vi "nanocal-frontend-18.vi"() -> ()   [LabVIEW 2018]
uses:
  nanocal - config.ctl
  resistoricicle.ctl
  channelicicle.ctl
  nanocal/Nanocalorimetry/data/MCL.lvlibp/SynkTek FPGA/FPGA_SharedResources/FPGASharedResources_Readings_ReadingChannelTypedef.ctl
  nanocal/Nanocalorimetry/data/MCL.lvlibp/SynkTek FPGA/FPGA_SharedResources/FPGASharedResources_Lockin_Typedef.ctl
  agregator -- action.ctl
  publisher action.ctl
  nanocal calc command.ctl
  copy of gyro pll V3 for LV18/cursor action.ctl
  linear interpolation iiii- complex.vi
  nanocal/Nanocalorimetry/data/NanoCalLib.lvlibp
  nanocal/Nanocalorimetry/data/MCL.lvlibp/SynkTek FPGA/FPGA_SharedResources/FPGA_SharedResources.lvlib
panel:
  in  "wait (ms)":u32=30
  in  "Stop":bool
  in  "Tab Control 2":enum32{"config", "read", "plots"}(tab)
  in  "nanocal config":T1={"Hs"={"out"=enum."D", "shunt R (Ohm)"=100000.0, "V"={"c"=enum."A V1", "l"=enum."Lock-in set L1"}, "\"I\""={"c"=enum."A V2", "l"=enum."Lock-in set L1"}}, "ofset heater"={"out"=enum."C", "\"I\""=enum."C V2", "shunt R (Ohm)"=10000.0}, "Ts"={"out"=enum."D", "shunt R (Ohm)"=100000.0, "V"={"c"=enum."D V1", "l"=enum."Lock-in set L1"}, "\"I\""={"c"=enum."D V2", "l"=enum."Lock-in set L1"}}, "Tr"={"out"=enum."B", "shunt R (Ohm)"=100000.0, "V"={"c"=enum."E V1", "l"=enum."Lock-in set L1"}, "\"I\""={"c"=enum."E V2", "l"=enum."Lock-in set L1"}}, "Hr"={"out"=enum."E", "shunt R (Ohm)"=100000.0, "V"={"c"=enum."B V1", "l"=enum."Lock-in set L1"}, "\"I\""={"c"=enum."B V2", "l"=enum."Lock-in set L1"}}, "differential"={"c"=enum."C V1", "l"=enum."Lock-in set L2"}} {"Hr"."shunt R (Ohm)" format="%#_6p"; "Tr"."shunt R (Ohm)" format="%#_6p"; "Ts"."shunt R (Ohm)" format="%#_6p"; "ofset heater"."shunt R (Ohm)" format="%#_6p"; "Hs"."shunt R (Ohm)" format="%#_6p"}
  out "diff":cluster{dbl[], dbl[]}[](graph)
  in  "history size":i32=10000
  out "C (J/K)":cluster{dbl[], dbl[]}[](graph)
  out "Ts":cluster{dbl[], dbl[]}[](graph)
  out "R(omega)":cluster{dbl[], dbl[]}[](graph)
  out "1/R(omega)":cluster{dbl[], dbl[]}[](graph)
  out "frequency (Hz)":dbl format="%#_3p"
  out "Cs (J/K)":dbl format="%#_3p"
  out "Ks (W/K)":dbl format="%#_3p"
  out "Hs -- \"I\" (V)":cdb format="%#_3p"
  out "Ts -- \"I\" (V)":cdb format="%#_3p"
  out "Ts":dbl format="%#_3p"
  # "Ts"
  # "Tr"
  # "Hs"
  # "Hr"
  # "offset heater"
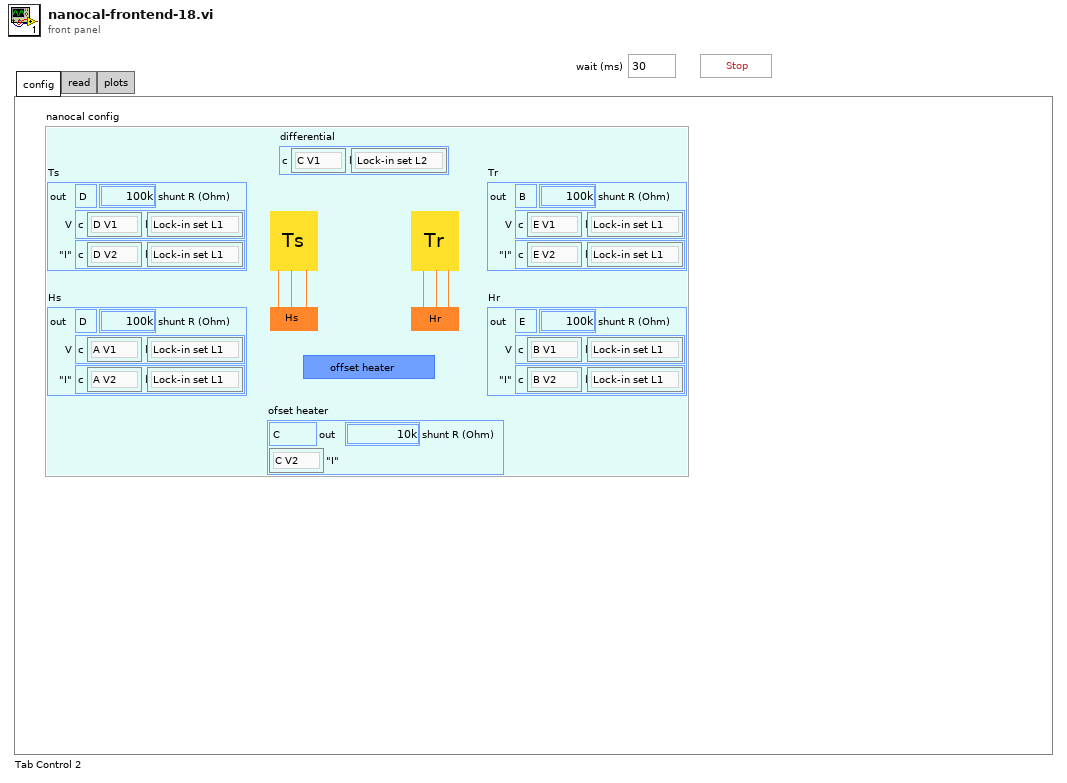
[diagram p1: front panel]
types:
  T1 = typedef "nanocal - config.ctl" = cluster{"Hs":T2, "ofset heater":cluster{"out":enum16{"A", "B", "C", "D", "E"}, "\"I\"":T4, "shunt R (Ohm)":dbl}, "Ts":T2, "Tr":T2, "Hr":T2, "differential":T3}
  T2 = typedef "resistoricicle.ctl" = cluster{"out":enum16{"A", "B", "C", "D", "E"}, "shunt R (Ohm)":dbl, "V":T3, "\"I\"":T3}
  T3 = typedef "channelicicle.ctl" = cluster{"c":T4, "l":T5}
  T4 = typedef "MCL.lvlibp/FPGA_SharedResources.lvlib/FPGASharedResources_Readings_ReadingChannelTypedef.ctl" = enum8{"A V1", "A V2", "B V1", "B V2", "C V1", "C V2", "D V1", "D V2", "E V1", "E V2", "A I", "B I", "C I", "D I", "E I", "Int."}
  T5 = typedef "MCL.lvlibp/FPGA_SharedResources.lvlib/FPGASharedResources_Lockin_Typedef.ctl" = enum8{"Lock-in set L1", "Lock-in set L2"}
  T6 = typedef "agregator -- action.ctl" = enum16{"append", "interpolate", "empty!", "force", "init", "scale", "read last"}
  T7 = typedef "MCL.lvlibp/MCL_DataRef.ctl" = refnum<vi>
  T8 = typedef "cursor action.ctl" = enum16{"range", "read", "write", "check", "zoom out", "smart zoom out", "zoom to aspect ratio 1", "zoom to win", "zoom out 20%", "zoom in 20%", "-empty", "smart zoom out&aspect", "move range left 20%", "move range right 20%", "move range up 20%", "move range down 20%", "zoom to X win", "zoom to Y win", "zoom out X", "zoom out Y", "zoom in X", "zoom in Y", "check plot scale"}
  T9 = typedef "nanocal calc command.ctl" = enum16{"void", "R(omega)", "C/T (J/K^2)"}
  T10 = typedef "publisher action.ctl" = enum16{"set", "get", "init", "check"}
  T11 = typedef "engine reading icicle.ctl" = cluster{"Ts -- V (V)":cdb, "Hr -- V (V)":cdb, "Hs -- V (V)":cdb, "Tr -- V (V)":cdb, "Diff -- V (V)":cdb, "offset (V)":cdb, "Ts -- \"I\" (V)":cdb, "Hs -- \"I\" (V)":cdb, "Tr -- \"I\" (V)":cdb, "Hr -- \"I\" (V)":cdb, "freq (Hz)":dbl}
  T12 = typedef "icicle.ctl" = cluster{"name":string, "units":string, "data":dbl}
  T13 = typedef "interpolation state - complex.ctl" = cluster{"requested size":i32, "Array":cdb[], "actual number of elements":i32}
  T14 = typedef "eventvkey.ctl" = enum16{"ASCII", "Enter", "Return", "Shift", "Ctrl", "Alt", "Cmd", "Opt", "Caps", "NumLock", "Clear", "Break", "Up", "Down", "Left", "Right", "Insert", "Delete", "Home", "End", "PageUp", "PageDown", "Escape", "Help", "Pause", "ScrollLock", "F1", "F2", "F3", "F4", "F5", "F6", "F7", "F8", "F9", "F10", "F11", "F12", "F13", "F14", "F15", "F16", "F17", "F18", "F19", "F20", "F21", "F22", "F23", "F24", "Play", "VolumeUp", "VolumeDown", "Mute", "Two Byte Char"}
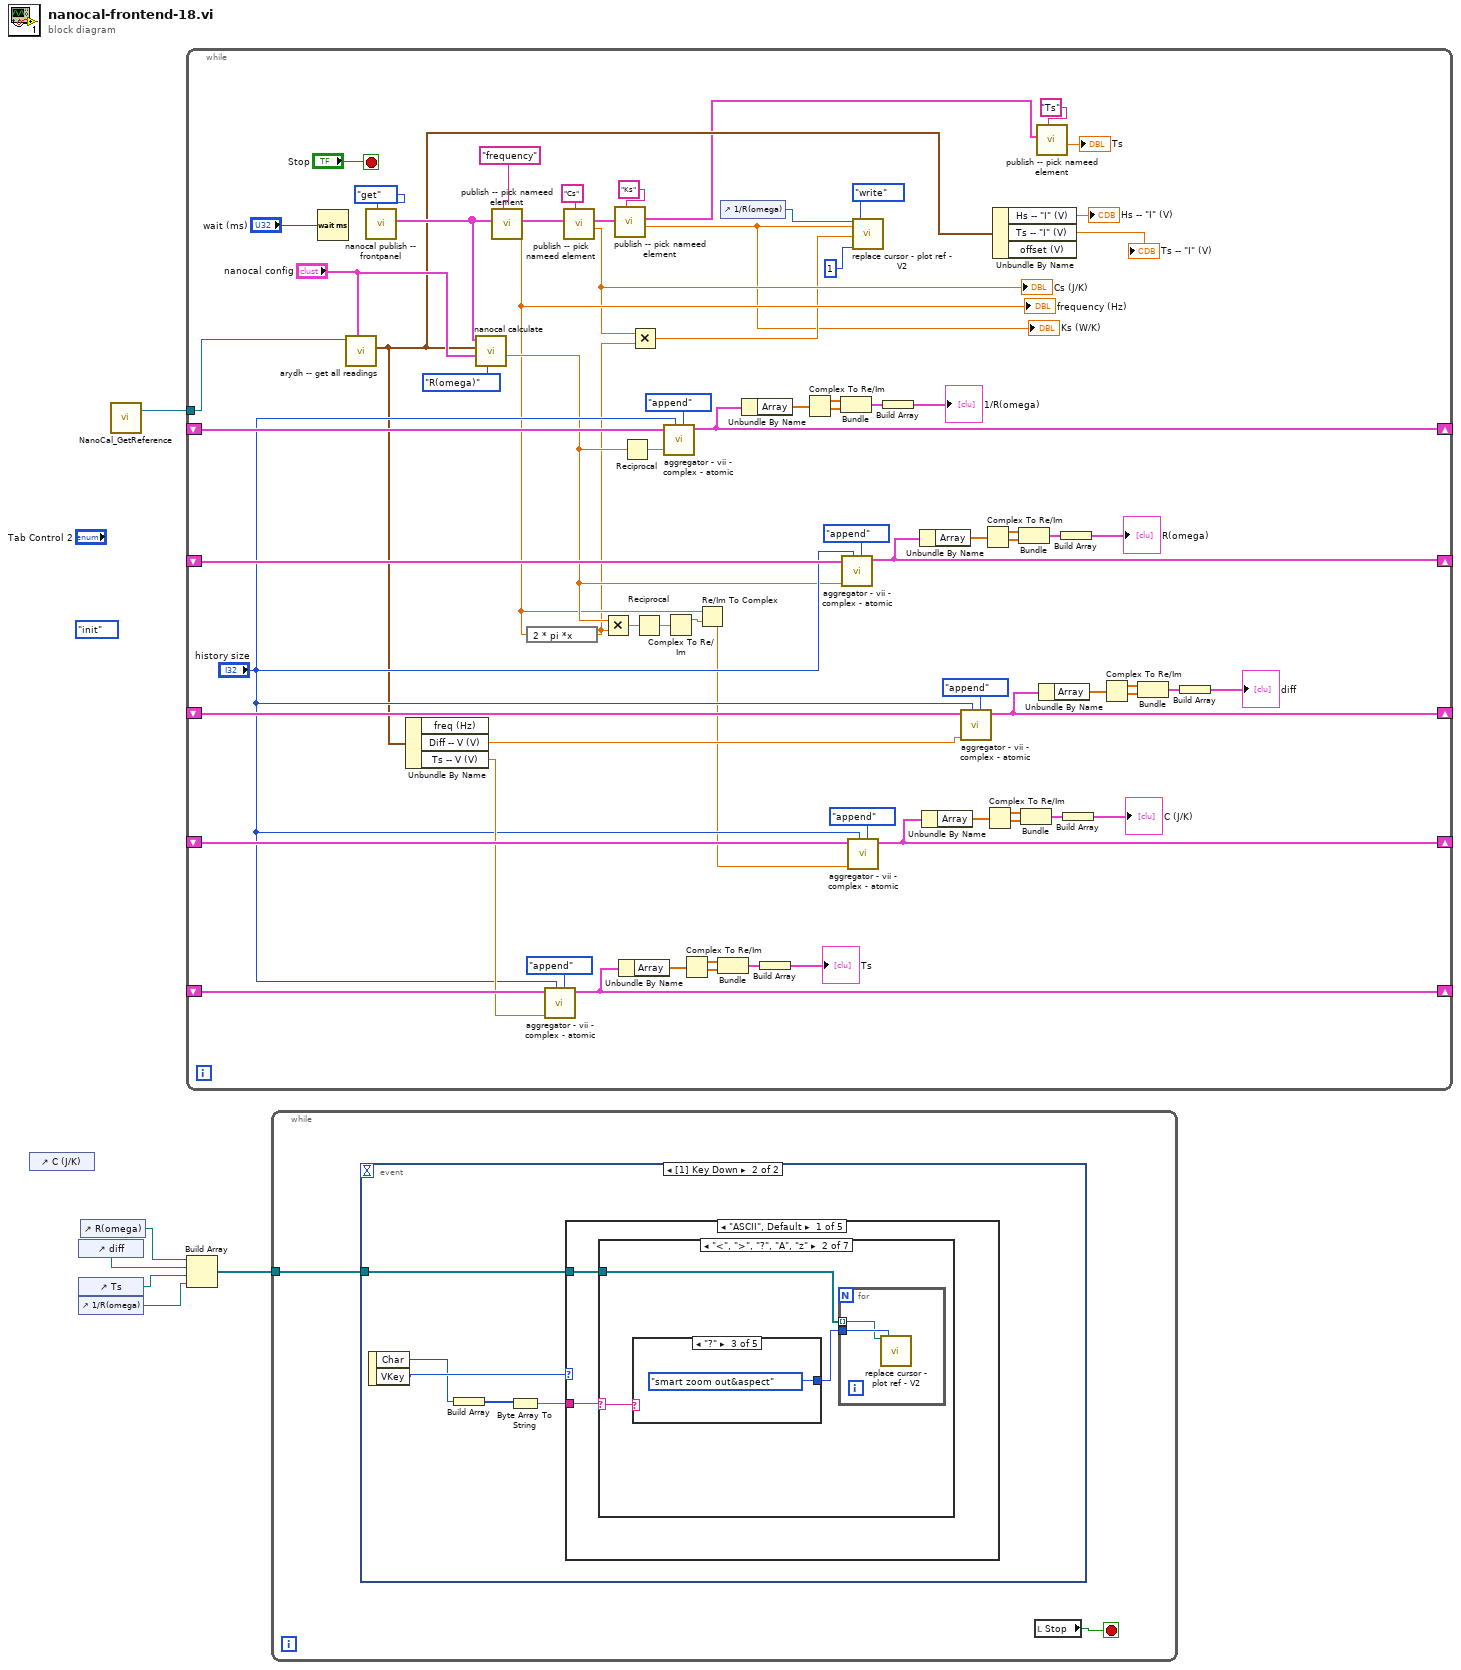
[diagram p0: block diagram]
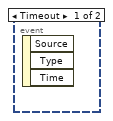
[diagram p2: hidden frame]
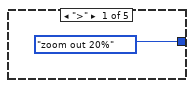
[diagram p4: hidden frame]
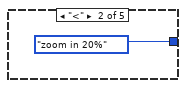
[diagram p5: hidden frame]
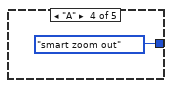
[diagram p6: hidden frame]
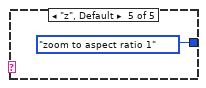
[diagram p7: hidden frame]
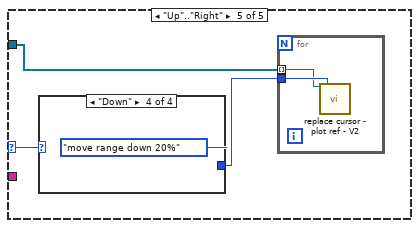
[diagram p16: hidden frame]
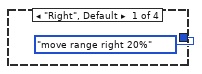
[diagram p17: hidden frame]
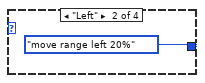
[diagram p18: hidden frame]
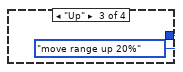
[diagram p19: hidden frame]
diagram:
  (unwired) agregator_--_action."init" ("aggregator action")
  n1 = control-ref of="C (J/K)"() -> ()  [unwired: 1 out]
  n2 = control-ref of="diff"() -> (w3:refnum<vi>)
  n3 = control-ref of="Ts"() -> (w4:refnum<vi>)
  n4 = control-ref of="1/R(omega)"() -> (w5:refnum<vi>)
  n5 = control-ref of="R(omega)"() -> (w1:refnum<vi>)
  n6 = call "NanoCal_GetReference.vi"() -> ("Connected MCL object"=w6:T7)  [unwired: 2 in, 1 out]
  n7 = while {
    tunnel: w6 -> [w47]
    shift-right: [w77] -> _
    shift-left: _ -> [w79]
    shift-right: [w65] -> _
    shift-left: _ -> [w64]
    shift-right: [w57] -> _
    shift-left: _ -> [w56]
    shift-right: [w49] -> _
    shift-left: _ -> [w48]
    shift-right: [w35] -> _
    shift-left: _ -> [w34]
    stop <- "Stop" stop-if-true
    n8 = Wait (ms)(milliseconds to wait="wait (ms)") -> ()  [unwired: 1 out]
    n9 = call "arydh -- get all readings.vi"("nanocal config"="nanocal config", "MCL object"=w47) -> ("engine reading"=w12:T11)  [unwired: 9 in]
    n10 = call "nanocal publish -- frontpanel.vi"("publisher action"=publisher_action."get") -> ("nanocal data array OUT"=w24:T12[])  [unwired: 10 in]
    n11 = Unbundle By Name(w12) -> ("Diff -- V (V)"=w46:cdb, "Ts -- V (V)"=w45:cdb)  [unwired: 1 out]
    n12 = call "nanocal calculate.vi"("nanocal calc command"=nanocal_calc_command."R(omega)", "nanocal config"="nanocal config", "engine reading"=w12, "nanocal data array"=w24) -> ("number"=w31:cdb)  [unwired: 7 in]
    n13 = call "publish -- pick nameed element.vi"("name"="frequency", "nanocal data array"=w24) -> ("element"=w26:dbl, "nanocal data array OUT"=w16:T12[])  [unwired: 8 in]
    "frequency (Hz)" <- w26
    n14 = expression code="2 * pi *x"(w26) -> (w22:dbl)
    n15 = call "aggregator - vii - complex - atomic.vi"("aggregator action"=agregator_--_action."append", "requested size"="history size", "number"=w45, "state IN"=w56) -> ("state OUT"=w57:T13)  [unwired: 4 in, 3 out]
    n16 = call "publish -- pick nameed element.vi"("name"="Cs", "nanocal data array"=w16) -> ("element"=w21:dbl, "nanocal data array OUT"=w23:T12[])  [unwired: 8 in]
    "Cs (J/K)" <- w21
    n17 = Multiply(x=w31, y=w22) -> (x*y=w30:cdb)
    n18 = call "publish -- pick nameed element.vi"("name"="Ks", "nanocal data array"=w23) -> ("element"=w19:dbl, "nanocal data array OUT"=w8:T12[])  [unwired: 8 in]
    "Ks (W/K)" <- w19
    n19 = Unbundle By Name(w57) -> ("Array"=w62:cdb[])
    n20 = Reciprocal(x=w31) -> (1/x=w32:cdb)
    n21 = Multiply(x=w21, y=w22) -> (x*y=w20:dbl)
    n22 = Reciprocal(x=w30) -> (1/x=w29:cdb)
    n23 = call "aggregator - vii - complex - atomic.vi"("aggregator action"=agregator_--_action."append", "requested size"="history size", "number"=w32, "state IN"=w34) -> ("state OUT"=w35:T13)  [unwired: 4 in, 3 out]
    n24 = Complex To Re/Im(x + iy=w29) -> (x=w28:dbl)  [unwired: 1 out]
    n25 = Complex To Re/Im(x + iy=w62) -> (x=w61:dbl[], y=w60:dbl[])
    n26 = Re/Im To Complex(1:w28, 2:w26) -> (0:w27:cdb)
    n27 = Bundle(w61, w60) -> (w59:cluster{dbl[], dbl[]})  [unwired: 1 in]
    n28 = control-ref of="1/R(omega)"() -> (w25:refnum<vi>)
    n29 = Unbundle By Name(w35) -> ("Array"=w40:cdb[])
    n30 = Build Array(w59) -> (→"Ts":cluster{dbl[], dbl[]}[])
    n31 = Complex To Re/Im(x + iy=w40) -> (x=w39:dbl[], y=w38:dbl[])
    n32 = Bundle(w39, w38) -> (w37:cluster{dbl[], dbl[]})  [unwired: 1 in]
    n33 = call "aggregator - vii - complex - atomic.vi"("aggregator action"=agregator_--_action."append", "requested size"="history size", "number"=w31, "state IN"=w48) -> ("state OUT"=w49:T13)  [unwired: 4 in, 3 out]
    n34 = call "aggregator - vii - complex - atomic.vi"("aggregator action"=agregator_--_action."append", "requested size"="history size", "number"=w27, "state IN"=w64) -> ("state OUT"=w65:T13)  [unwired: 4 in, 3 out]
    n35 = call "replace cursor - plot ref - V2.vi"("Plot ref in"=w25, "new X"=w19, "new  Y"=w20, "cursor index"=1, "cursor action"=cursor_action."write") -> ()  [unwired: 11 in, 4 out]
    n36 = Build Array(w37) -> (→"1/R(omega)":cluster{dbl[], dbl[]}[])
    n37 = Unbundle By Name(w49) -> ("Array"=w54:cdb[])
    n38 = Unbundle By Name(w65) -> ("Array"=w70:cdb[])
    n39 = call "aggregator - vii - complex - atomic.vi"("aggregator action"=agregator_--_action."append", "requested size"="history size", "number"=w46, "state IN"=w79) -> ("state OUT"=w77:T13)  [unwired: 4 in, 3 out]
    n40 = Complex To Re/Im(x + iy=w54) -> (x=w53:dbl[], y=w52:dbl[])
    n41 = Complex To Re/Im(x + iy=w70) -> (x=w69:dbl[], y=w68:dbl[])
    n42 = Unbundle By Name(w12) -> ("Hs -- \"I\" (V)"=→"Hs -- \"I\" (V)":cdb, "Ts -- \"I\" (V)"=→"Ts -- \"I\" (V)":cdb)  [unwired: 1 out]
    n43 = Bundle(w53, w52) -> (w51:cluster{dbl[], dbl[]})  [unwired: 1 in]
    n44 = Bundle(w69, w68) -> (w67:cluster{dbl[], dbl[]})  [unwired: 1 in]
    n45 = call "publish -- pick nameed element.vi"("name"="Ts", "nanocal data array"=w8) -> ("element"=→"Ts":dbl)  [unwired: 8 in, 1 out]
    n46 = Unbundle By Name(w77) -> ("Array"=w76:cdb[])
    n47 = Build Array(w51) -> (→"R(omega)":cluster{dbl[], dbl[]}[])
    n48 = Build Array(w67) -> (→"C (J/K)":cluster{dbl[], dbl[]}[])
    n49 = Complex To Re/Im(x + iy=w76) -> (x=w75:dbl[], y=w74:dbl[])
    n50 = Bundle(w75, w74) -> (w73:cluster{dbl[], dbl[]})  [unwired: 1 in]
    n51 = Build Array(w73) -> (→"diff":cluster{dbl[], dbl[]}[])
  }
  n52 = Build Array(w1, w3, w4, w5) -> (w2:refnum<vi>[])
  n53 = while {
    tunnel: w2 -> [w82]
    stop <- w83 stop-if-true
    n54 = event shown="[1] Key Down" {
      selector: _ -> [_ _]
      dyn-events: _ -> [_ _]
      timeout: _ -> [_ _]
      tunnel: w82 -> [_ w84]
      event Timeout {
        n55 = event-data() -> ()  [unwired: 1 in, 3 out]
      }
      event Key Down {
        n56 = event-data() -> ("Char"=w85:i16, "VKey"=w87:T14)  [unwired: 1 in]
        n57 = Build Array(w85) -> (w86:i16[])
        n58 = Byte Array To String(unsigned byte array=w86) -> (string=w88:string)
        n59 = case shown="\"ASCII\", Default" w87 {
          selector: w87 -> [_ _ _ _ w103]
          tunnel: w88 -> [w90 _ _ _ _]
          tunnel: w84 -> [w89 _ _ _ w101]
          frame "ASCII", Default {
            n60 = case shown="\"<\", \">\", \"?\", \"A\", \"z\"" w90 {
              selector: w90 -> [_ w93 _ _ _ _ _]
              tunnel: w89 -> [_ w92 _ _ _ _ _]
              frame "0", Default {
              }
              frame "<", ">", "?", "A", "z" {
                n61 = case shown="\"?\"" w93 {
                  tunnel: [cursor_action."zoom out 20%" ("cursor action") cursor_action."zoom in 20%" ("cursor action") cursor_action."smart zoom out&aspect" ("cursor action") cursor_action."smart zoom out" ("cursor action") cursor_action."zoom to aspect ratio 1" ("cursor action")] -> w91
                  frame ">" {
                  }
                  frame "<" {
                  }
                  frame "?" {
                  }
                  frame "A" {
                  }
                  frame "z", Default {
                  }
                }
                n62 = for {
                  tunnel: w91 -> [w95]
                  tunnel: w92 -> [w94] mode=indexing
                  n63 = call "replace cursor - plot ref - V2.vi"("Plot ref in"=w94, "cursor action"=w95) -> ()  [unwired: 14 in, 4 out]
                }
              }
              frame "r" {
              }
              frame "'", ";", "[", "]", "{", "}" {
              }
              frame "@" {
              }
              frame "#" {
              }
              frame "q" {
              }
            }
          }
          frame "Escape" {
          }
          frame "PageUp" {
          }
          frame "PageDown" {
          }
          frame "Up".."Right" {
            n64 = case shown="\"Down\"" w103 {
              tunnel: [cursor_action."move range right 20%" ("cursor action") cursor_action."move range left 20%" ("cursor action") cursor_action."move range up 20%" ("cursor action") cursor_action."move range down 20%" ("cursor action")] -> w102
              frame "Right", Default {
              }
              frame "Left" {
              }
              frame "Up" {
              }
              frame "Down" {
              }
            }
            n65 = for {
              tunnel: w102 -> [w105]
              tunnel: w101 -> [w104] mode=indexing
              n66 = call "replace cursor - plot ref - V2.vi"("Plot ref in"=w104, "cursor action"=w105) -> ()  [unwired: 14 in, 4 out]
            }
          }
        }
      }
    }
    n67 = local read "Stop"() -> (w83:bool)
  }
